vi "CompareDialog.vi"(9 "RegEx":string, 11 "Match":string) -> ()   [LabVIEW 2022 SP3, in "MES_Local.lvlib" / "MES_Local.lvclass"]
uses:
  MES_Local.lvclass
panel:
  in  "OK Button":bool
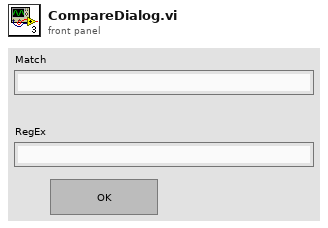
[diagram p1: front panel]
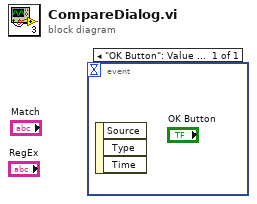
[diagram p0: block diagram]
diagram:
  n1 = event shown="[0] \"OK Button\": Value Change" {
    selector: _ -> [_]
    dyn-events: _ -> [_]
    timeout: _ -> [_]
    event "OK Button": Value Change {
      n2 = event-data() -> ()  [unwired: 1 in, 3 out]
    }
  }
